vi "LVFunction_Imop_CameraFile_GetFocal.vi"(0 "Configuration file path":path, 11 "error in (no error)":errorcluster) -> (4 "Configuration file path (dup)":path, 6 "Focal":u8, 15 "error out":errorcluster)   [LabVIEW 2020]
doc: "Get acquisition information from image file.\n\n--------------------------------------------------------------------------------\n\n<B>image_file_pathIn</B> : Absolute path to image file.\n<B>image_file_pathOut</B> : Absolute path to image file.\n<B>bit_depth</B> : Image bits depth.\n<B>size</B> : Image size.\n<B>time_stamp</B> : Acquisition time.\n<B>haso_serial_number</B> : Haso serial number.\n<B>camera_serial_number</B> : Camera serial number.\n<B>em_ccd_gain</B> : Emccd gain.\n<B>nb_summed_images</B> : Number summed image.\n<B>exposure_time_requested</B> : Exposure duration requested (us).\n<B>exposure_time_applied</B> : Exposure duration applied (us).\n<B>ErrorIn</B> : Error\n<B>ErrorOut</B> : Error\n\n--------------------------------------------------------------------------------"
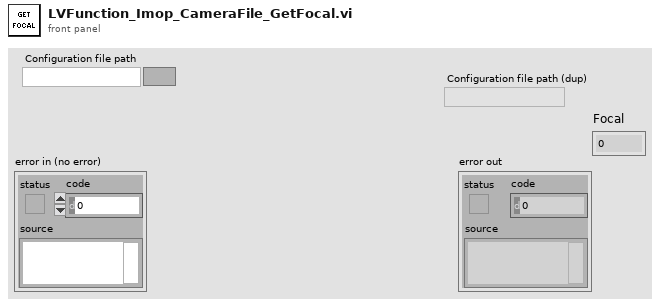
[diagram p1: front panel]
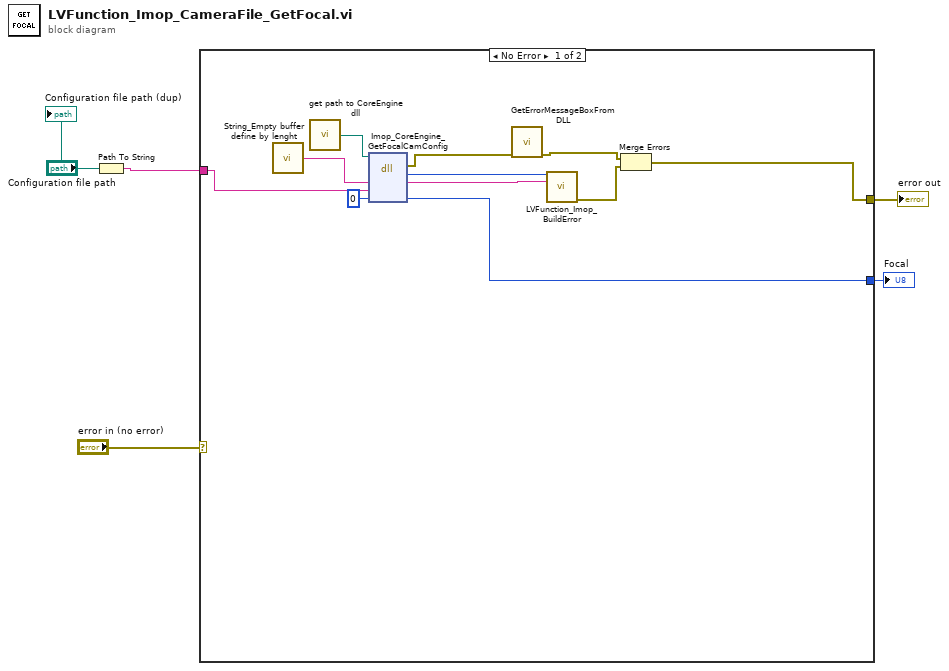
[diagram p0: block diagram]
diagram:
  n1 = Path To String(path="Configuration file path") -> (string=w3:string)
  n2 = case shown="No Error" "error in (no error)" {
    selector: "error in (no error)" -> [_ w17]
    tunnel: [w8 w17] -> w4
    tunnel: w3 -> [w12 _]
    tunnel: [w6 _] -> w1
    frame No Error {
      n3 = call "String_Empty buffer define by lenght.vi"() -> ("Empty buffer"=w11:string)  [unwired: 1 in]
      n4 = call "get path to CoreEngine dll.vi"() -> ("path to c_interface_vc100.dll"=w14:path)  [unwired: 12 in, 3 out]
      n5 = dll-call lib="D:/FLE/0.Code/CoreEngine4_Suite/LV2011_interface/DLLs/c_interface_vc100.dll" fn="Imop_CoreEngine_GetFocalCamConfig"(path in=w14, "message"=w11, "path"=w12, "Focal"=u8 0) -> (error out=w13:errorcluster, "return type"=w16:i32, "message"=w15:string, "Focal"=w6:u8)  [unwired: 3 in, 1 out]
      n6 = call "GetErrorMessageBoxFromDLL.vi"("error IN"=w13) -> ("error OUT"=w10:errorcluster)  [unwired: 10 in]
      n7 = call "LVFunction_Imop_BuildError.vi"("code"=w16, "String to Prepend to source (\"\")"=w15) -> ("error out"=w9:errorcluster)  [unwired: 13 in]
      n8 = Merge Errors(w10, w9) -> (w8:errorcluster)
    }
    frame Error {
    }
  }
  "error out" <- w4
  "Focal" <- w1
  "Configuration file path (dup)" <- "Configuration file path"
